vi "Begin.vi"() -> (0 "error out":errorcluster)   [LabVIEW 2013]
doc: "Called before other user functions, this VI is expected to open initial I/O refnums, load in file data, and do all program initialization. Notice that the <B>error out</B> terminal is simply used for data flow. Wiring it to other structures or subVIs ensures that this VI runs first."
uses:
  <vilib>/Rock Robotics/WPI/DriverStation/WPI_DriverStationRobotMode2.ctl
  <vilib>/Rock Robotics/WPI/Joystick/WPI_JoystickDeviceEnum.ctl
  <vilib>/Rock Robotics/WPI/SafetyOutput/WPI_SafetyOutputConfigMenu.ctl
  <vilib>/Rock Robotics/WPI/CAN/Jaguar/SubVIs/WPI_CANJaguar_ControlMode.ctl
  <vilib>/Rock Robotics/WPI/CAN/Jaguar/SubVIs/WPI_CANJaguar_PositionReference.ctl
  Robot Global Data.vi
  <vilib>/Utility/config.llb/Read Key (Double).vi
  <vilib>/Utility/config.llb/Read Key (String).vi
  <vilib>/Rock Robotics/WPI/MotorControl/WPI_MotorControlOpen Jaguar.vi
  <vilib>/Rock Robotics/WPI/RobotDrive/WPI_RobotDriveOpen4MotorWithCANJaguar.vi
  <vilib>/Rock Robotics/WPI/MotorControl/WPI_MotorControlOpenCANJaguar.vi
  <vilib>/Rock Robotics/SystemInterfaces/Typedef/FPGA_TypedefDigitalModule.ctl
  <vilib>/Utility/config.llb/NI_LVConfig.lvlib
  <vilib>/Rock Robotics/WPI/Solenoid/WPI_SolenoidChannel.ctl
  <vilib>/Rock Robotics/SystemInterfaces/DIO/FPGA_DIOChannel.ctl
  <vilib>/Rock Robotics/SystemInterfaces/DIO/FPGA_DIORelayChannel.ctl
  <vilib>/Rock Robotics/WPI/Solenoid/WPI_SolenoidOpenSingle.vi
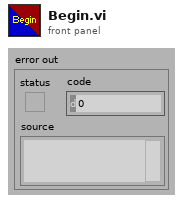
[diagram p1: front panel]
types:
  T1 = typedef "WPI_SafetyOutputConfigMenu.ctl" = enum16{"Enable", "Disable"}
  T2 = typedef "WPI_JoystickDeviceEnum.ctl" = enum16{"USB 1", "USB 2", "USB 3", "USB 4", "Kinect 1", "Kinect 2"}
  T3 = cluster{"Left Motor Positions":cluster{"Low Extreme - 0 Degrees":dbl, "High Extreme - 180 Degrees":dbl}, "Right Motor Positions":cluster{"Low Extreme - 0 Degrees":dbl, "High Extreme - 180 Degrees":dbl}}
  T4 = cluster{"Low Extreme - 0 Degrees":dbl, "High Extreme - 180 Degrees":dbl}
  T5 = typedef "WPI_DriverStationRobotMode2.ctl" = enum16{"Autonomous Disabled", "Autonomous Enabled", "Teleop Disabled", "Teleop Enabled", "Timeout", "Finish", "Test Disabled", "Test Enabled"}
  T6 = typedef "NI_LVConfig.lvlib/Config Data RefNum.ctl" = refnum<k1>
  T7 = typedef "WPI_RobotDriveDevRef.ctl" = cluster{"DevStatus":errorcluster, "Motors[]":T8[], "Square Inputs":bool, "Max Output":dbl, "Isochronous":bool}
  T8 = typedef "WPI_MotorControlDeviceRef.ctl" = cluster{"DeviceStatus":errorcluster, "Type":enum16{"PWM", "CAN"}, "PWM":cluster{"Digital Module":T9, "PWM Channel":T10, "DeadBand":T11}, "CAN":cluster{"Device Number":u8, "Control Mode":T12, "Semaphore":T13, "Max Vout":dbl}, "Invert":bool, "TransformRef":T14, "InvTransformRef":T14}
  T9 = typedef "FPGA_TypedefDigitalModule.ctl" = enum16{"Digital Module 1", "Digital Module 2"}
  T10 = typedef "FPGA_DIOPWMChannel.ctl" = enum8{"PWM 1", "PWM 2", "PWM 3", "PWM 4", "PWM 5", "PWM 6", "PWM 7", "PWM 8", "PWM 9", "PWM 10", "Invalid"}
  T11 = typedef "WPI_PWMDeadband.ctl" = cluster{"Name":string, "maxPositivePwm":i32, "minPositivePwm":i32, "centerPwm":i32, "maxNegativePwm":i32, "minNegativePwm":i32, "angularRange":u16}
  T12 = typedef "WPI_CANJaguar_ControlMode.ctl" = enum8{"Percent VBus", "Current", "Speed", "Position", "Voltage"}
  T13 = typedef "Semaphore RefNum" = refnum<k1>
  T14 = typedef "WPI_PWMTransform_ConPane.ctl" = refnum<vi>
  T15 = typedef "FPGA_DIORelayChannel.ctl" = enum8{"Relay 1", "Relay 2", "Relay 3", "Relay 4", "Relay 5", "Relay 6", "Relay 7", "Relay 8", "Invalid"}
  T16 = typedef "FPGA_DIOChannel.ctl" = enum8{"DIO 1", "DIO 2", "DIO 3", "DIO 4", "DIO 5", "DIO 6", "DIO 7", "DIO 8", "DIO 9", "DIO 10", "DIO 11", "DIO 12", "DIO 13", "DIO 14", "Invalid"}
  T17 = typedef "WPI_SolenoidChannel.ctl" = enum8{"Solenoid 1", "Solenoid 2", "Solenoid 3", "Solenoid 4", "Solenoid 5", "Solenoid 6", "Solenoid 7", "Solenoid 8", "Invalid"}
  T18 = typedef "WPI_SolenoidDevRef.ctl" = cluster{"DevStatus":errorcluster, "Solenoid Module":T19, "Forward Solenoid Channel":T17, "Reverse Solenoid Channel":T17}
  T19 = typedef "FPGA_TypedefSolenoidModule.ctl" = enum16{"Solenoid Module 1", "Solenoid Module 2"}
  T20 = typedef "WPI_CompressorDevRef.ctl" = cluster{"DevStatus":errorcluster, "DigitalInputDevRef":T21, "RelayDevRef":T22}
  T21 = typedef "WPI_DigitalInputDevRef.ctl" = cluster{"DevStatus":errorcluster, "DIO Channel":T16, "Digital Module":T9}
  T22 = typedef "WPI_RelayDevRef.ctl" = cluster{"DevStatus":errorcluster, "Relay Channel":T15, "Digital Module":T9, "Relay Direction":T23}
  T23 = typedef "WPI_RelayDirection.ctl" = enum16{"Both directions", "Forward only", "Reverse only"}
  T24 = typedef "WPI_CANJaguar_PositionReference.ctl" = u8
  T25 = typedef "WPI_JoystickDevRef.ctl" = cluster{"Device":T2}
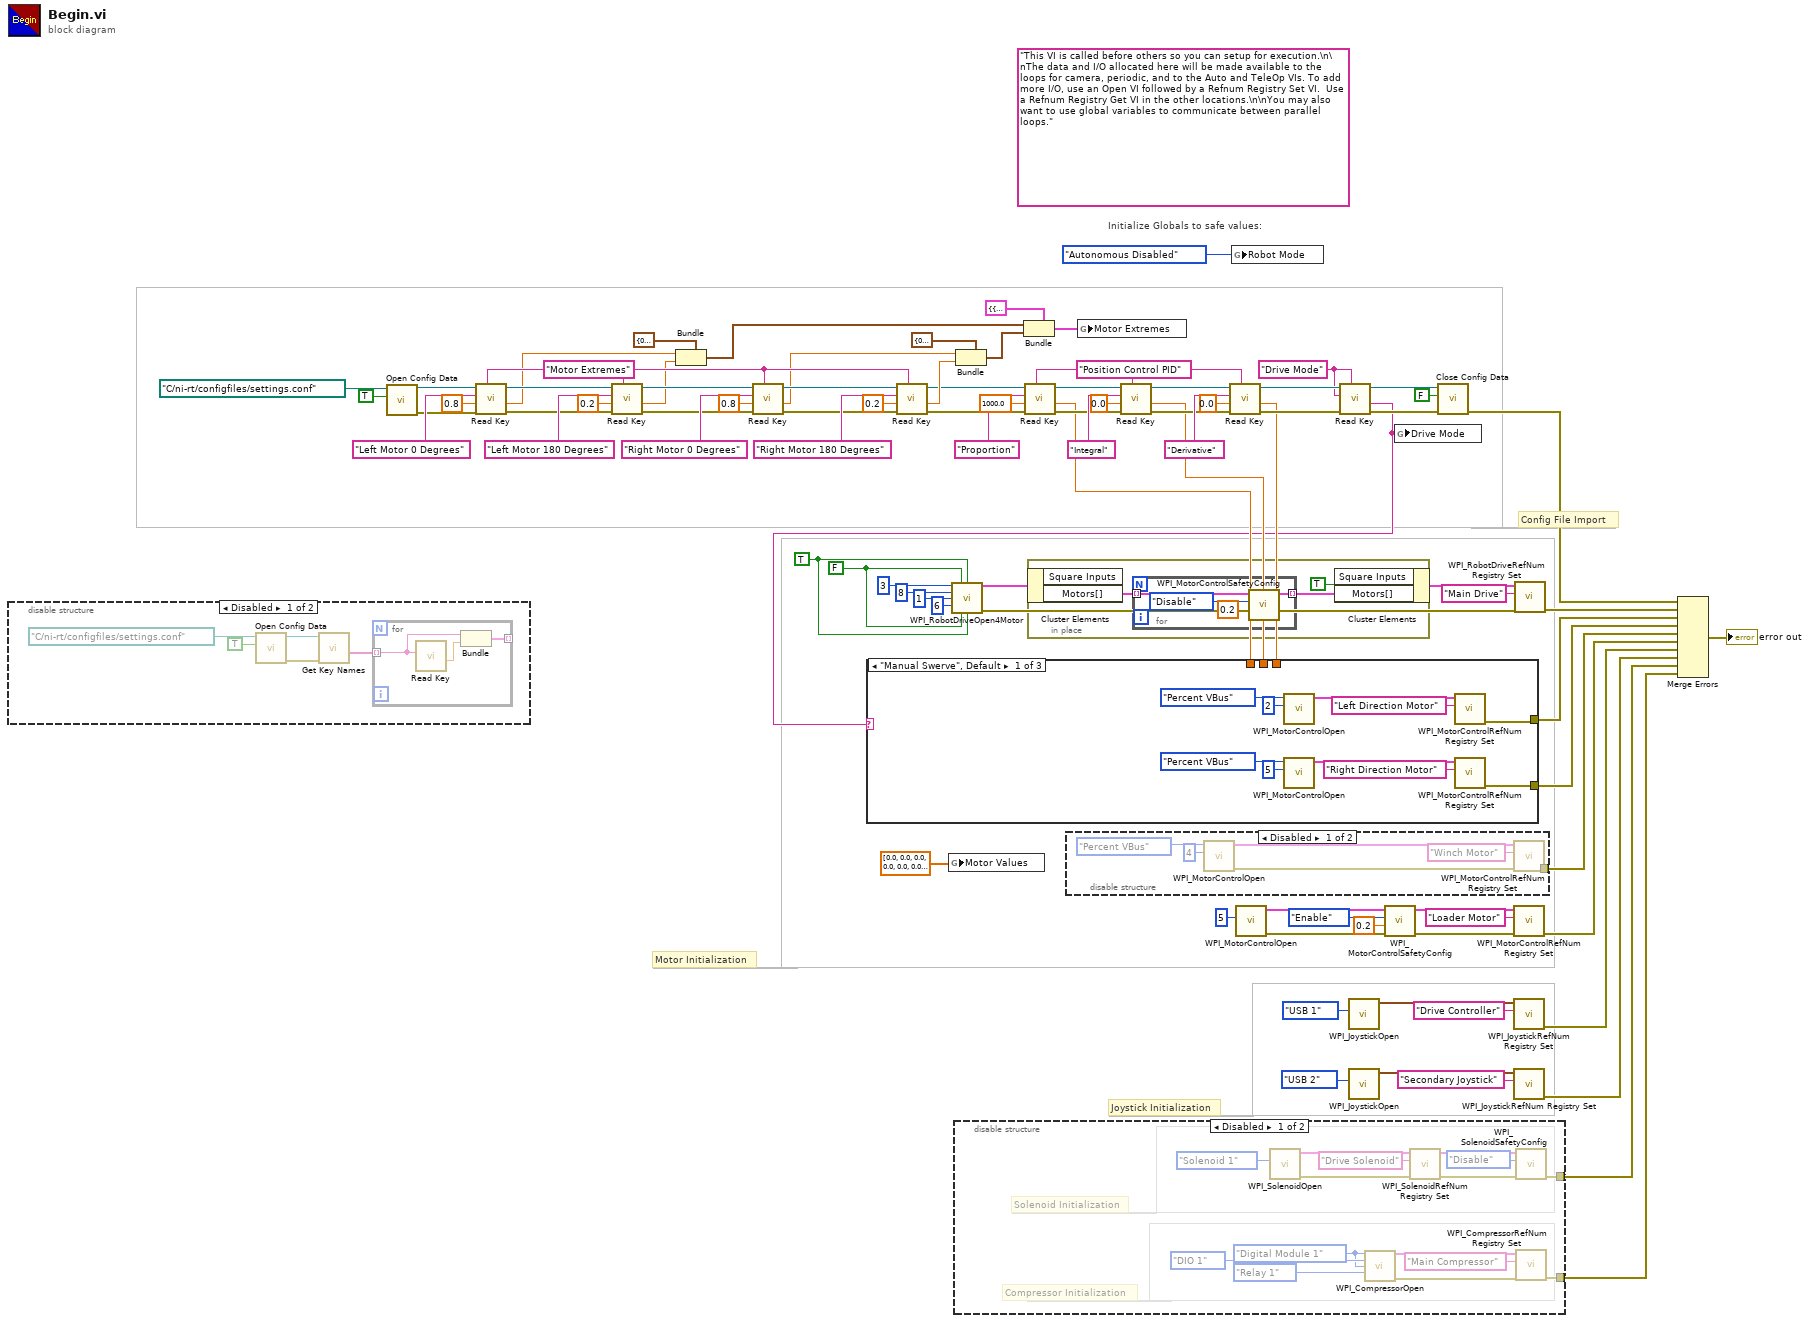
[diagram p0: block diagram]
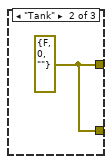
[diagram p5: hidden frame]
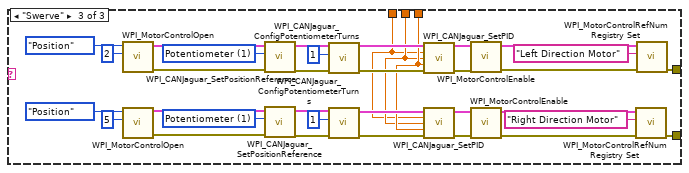
[diagram p6: hidden frame]
diagram:
  w1 = TRUE ("Rear Right Motor Inverted")
  w2 = FALSE
  w27 = "Drive Mode" ("section")
  w56 = "Position Control PID" ("section")
  w70 = "Motor Extremes" ("section")
  (unwired) "This VI is called before others so you can setup for execution.\n\nThe data and I/O allocated here will be made available to the loops for camera, periodic, and to the Auto and TeleOp VIs. To add more I/O, use an Open VI followed by a Refnum Registry Set VI.  Use a Refnum Registry Get VI in the other locations.\n\nYou may also want to use global variables to communicate between parallel loops."
  # "Config File Import"
  # "Joystick Initialization"
  # "Motor Initialization"
  # "Initialize Globals to safe values:"
  n1 = disable-structure shown="Disabled" {
    frame Disabled {
      n2 = call <vilib>:"Open Config Data.vi"("create file if necessary (T)"=TRUE, "configuration file path"=path "C:/ni-rt/configfiles/settings.conf") -> ("error out"=w91:errorcluster, "refnum"=w92:T6)  [unwired: 7 in, 1 out]
      n3 = call <vilib>:"Get Key Names.vi"("error in (no error)"=w91, "refnum"=w92) -> ("key names"=w90:string[])  [unwired: 6 in, 3 out]
      n4 = for {
        tunnel: w90 -> [w97] mode=indexing
        tunnel: [w95] -> _ mode=indexing
        n5 = call-poly <vilib>:"Read Key.vi"("key"=w97) -> ("value"=w96:dbl)  [unwired: 7 in, 3 out]
        n6 = Bundle("String"=w97, "value"=w96) -> (w95:cluster{"String":string, "value":dbl})  [unwired: 1 in]
      }
    }
    frame Enabled {
    }
  }
  n7 = call <vilib>:"Open Config Data.vi"("create file if necessary (T)"=TRUE, "configuration file path"=path "C:/ni-rt/configfiles/settings.conf") -> ("error out"=w34:errorcluster, "refnum"=w83:T6)  [unwired: 7 in, 1 out]
  n8 = call-poly <vilib>:"Read Key.vi"("section"=w70, "error in (no error)"=w34, "default value"=0.8, "key"="Left Motor 0 Degrees", "refnum"=w83) -> ("error out"=w35:errorcluster, "value"=w55:dbl, "refnum out"=w78:T6)  [unwired: 3 in, 1 out]
  n9 = call-poly <vilib>:"Read Key.vi"("section"=w70, "error in (no error)"=w35, "default value"=0.2, "key"="Left Motor 180 Degrees", "refnum"=w78) -> ("error out"=w36:errorcluster, "value"=w54:dbl, "refnum out"=w72:T6)  [unwired: 3 in, 1 out]
  n10 = Bundle(cluster=T4 {"Low Extreme - 0 Degrees"=0.0, "High Extreme - 180 Degrees"=0.0} ("Left Motor Positions"), "Low Extreme - 0 Degrees"=w55, "High Extreme - 180 Degrees"=w54) -> (w65:T4)
  n11 = call-poly <vilib>:"Read Key.vi"("section"=w70, "error in (no error)"=w36, "default value"=0.8, "key"="Right Motor 0 Degrees", "refnum"=w72) -> ("error out"=w37:errorcluster, "value"=w53:dbl, "refnum out"=w73:T6)  [unwired: 3 in, 1 out]
  n12 = call-poly <vilib>:"Read Key.vi"("section"=w70, "error in (no error)"=w37, "default value"=0.2, "key"="Right Motor 180 Degrees", "refnum"=w73) -> ("error out"=w38:errorcluster, "value"=w52:dbl, "refnum out"=w51:T6)  [unwired: 3 in, 1 out]
  n13 = global write "Robot Global Data.vi" "Motor Values"(dbl[] [0.0, 0.0, 0.0, 0.0, 0.0, 0.0, 0.0, 0.0]) -> ()
  n14 = call-poly <vilib>:"WPI_RobotDriveOpen4Motor.vi"("Rear Left Motor"=u8 3, "Rear Left Motor Inverted"=w2, "Rear Right Motor Inverted"=w1, "Rear Right Motor"=u8 8, "Front Left Motor"=u8 1, "Front Right Motor"=u8 6, "Front Left Motor Inverted"=w2, "Front Right Motor Inverted"=w1) -> ("RobotDriveDevRef"=w49:T7, "error out"=w41:errorcluster)  [unwired: 6 in]
  n15 = disable-structure shown="Disabled" {
    disable-tunnel: [w105 _] -> w24
    disable-tunnel: [w104 _] -> w20
    frame Disabled {
      w99 = FPGA_TypedefDigitalModule."Digital Module 1" ("Pressure Switch Digital Module (Module 1)")
      # "Compressor Initialization"
      # "Solenoid Initialization"
      n16 = call-poly <vilib>:"WPI_SolenoidOpen.vi"("Solenoid Channel"=WPI_SolenoidChannel."Solenoid 1") -> ("error out"=w111:errorcluster, "SolenoidDevRef"=w112:T18)  [unwired: 9 in]
      n17 = call <vilib>:"WPI_CompressorOpen.vi"("Pressure Switch Digital Module (Module 1)"=w99, "Pressure Switch DIO Channel"=FPGA_DIOChannel."DIO 1", "Relay Digital Module (Module 1)"=w99, "Relay Channel"=FPGA_DIORelayChannel."Relay 1") -> ("CompressorDevRef"=w103:T20, "error out"=w98:errorcluster)  [unwired: 10 in]
      n18 = call <vilib>:"WPI_SolenoidRefNum Registry Set.vi"("error in (no error)"=w111, "refnum name"="Drive Solenoid", "SolenoidDevRef"=w112) -> ("error out"=w109:errorcluster, "SolenoidDevRef"=w110:T18)  [unwired: 7 in]
      n19 = call <vilib>:"WPI_SolenoidSafetyConfig.vi"("error in (no error)"=w109, "mode"=WPI_SafetyOutputConfigMenu."Disable", "SolenoidDevRef"=w110) -> ("error out"=w105:errorcluster)  [unwired: 7 in, 1 out]
      n20 = call <vilib>:"WPI_CompressorRefNum Registry Set.vi"("error in (no error)"=w98, "refnum name"="Main Compressor", "CompressorDevRef"=w103) -> ("error out"=w104:errorcluster)  [unwired: 7 in, 1 out]
    }
    frame Enabled {
    }
  }
  n21 = Bundle(cluster=T4 {"Low Extreme - 0 Degrees"=0.0, "High Extreme - 180 Degrees"=0.0} ("Right Motor Positions"), "Low Extreme - 0 Degrees"=w53, "High Extreme - 180 Degrees"=w52) -> (w66:T4)
  n22 = Bundle(cluster=T3 {"Left Motor Positions"={"Low Extreme - 0 Degrees"=0.0, "High Extreme - 180 Degrees"=0.0}, "Right Motor Positions"={"Low Extreme - 0 Degrees"=0.0, "High Extreme - 180 Degrees"=0.0}} ("Motor Extremes"), "Left Motor Positions"=w65, "Right Motor Positions"=w66) -> (w50:T3)
  n23 = call-poly <vilib>:"Read Key.vi"("section"=w56, "error in (no error)"=w38, "default value"=1000.0, "key"="Proportion", "refnum"=w51) -> ("error out"=w39:errorcluster, "value"=w17:dbl, "refnum out"=w60:T6)  [unwired: 3 in, 1 out]
  n24 = in-place {
    n25 = in-place-cluster #1(w49) -> ("Motors[]"=w114:T8[])  [unwired: 1 out]
    n26 = for {
      tunnel: w114 -> [w119] mode=indexing
      tunnel: [w118] -> w113 mode=indexing
      n27 = call <vilib>:"WPI_MotorControlSafetyConfig.vi"("timeout (s)"=0.2, "mode"=WPI_SafetyOutputConfigMenu."Disable", "MotorControlDevRef"=w119) -> ("MotorControlDevRef"=w118:T8)  [unwired: 7 in, 1 out]
    }
    n28 = in-place-cluster #1("Square Inputs"=TRUE, "Motors[]"=w113) -> (w48:T7)
  }
  n29 = disable-structure shown="Disabled" {
    disable-tunnel: [w120 _] -> w32
    frame Disabled {
      n30 = call-poly <vilib>:"WPI_MotorControlOpen.vi"("Device Number"=u8 4, "Control Mode"=WPI_CANJaguar_ControlMode."Percent VBus") -> ("error out"=w121:errorcluster, "MotorControlDeviceRef"=w122:T8)  [unwired: 8 in]
      n31 = call <vilib>:"WPI_MotorControlRefNum Registry Set.vi"("error in (no error)"=w121, "refnum name"="Winch Motor", "MotorControlDevRef"=w122) -> ("error out"=w120:errorcluster)  [unwired: 7 in, 1 out]
    }
    frame Enabled {
    }
  }
  n32 = global write "Robot Global Data.vi" "Motor Extremes"(w50) -> ()
  n33 = call-poly <vilib>:"Read Key.vi"("section"=w56, "error in (no error)"=w39, "default value"=0.0, "key"="Integral", "refnum"=w60) -> ("error out"=w40:errorcluster, "value"=w18:dbl, "refnum out"=w57:T6)  [unwired: 3 in, 1 out]
  n34 = call-poly <vilib>:"Read Key.vi"("section"=w56, "error in (no error)"=w40, "default value"=0.0, "key"="Derivative", "refnum"=w57) -> ("error out"=w30:errorcluster, "value"=w19:dbl, "refnum out"=w31:T6)  [unwired: 3 in, 1 out]
  n35 = global write "Robot Global Data.vi" "Robot Mode"(WPI_DriverStationRobotMode2."Autonomous Disabled" ("Robot Mode")) -> ()
  n36 = call-poly <vilib>:"WPI_MotorControlOpen.vi"("PWM Channel"=u8 5 ("Device Number")) -> ("error out"=w7:errorcluster, "MotorControlDeviceRef"=w10:T8)  [unwired: 9 in]
  n37 = call-poly <vilib>:"Read Key.vi"("section"=w27, "error in (no error)"=w30, "key"=w27, "refnum"=w31) -> ("error out"=w29:errorcluster, "value"=w14:string, "refnum out"=w28:T6)  [unwired: 4 in, 1 out]
  n38 = case shown="\"Manual Swerve\", Default" w14 {
    tunnel: [w126 w136 w141] -> w16
    tunnel: [w127 w136 w140] -> w15
    tunnel: w19 -> [_ _ w139]
    tunnel: w18 -> [_ _ w138]
    tunnel: w17 -> [_ _ w137]
    frame "Manual Swerve", Default {
      n39 = call-poly <vilib>:"WPI_MotorControlOpen.vi"("Device Number"=u8 2, "Control Mode"=WPI_CANJaguar_ControlMode."Percent VBus") -> ("MotorControlDeviceRef"=w130:T8)  [unwired: 8 in, 1 out]
      n40 = call-poly <vilib>:"WPI_MotorControlOpen.vi"("Device Number"=u8 5, "Control Mode"=WPI_CANJaguar_ControlMode."Percent VBus") -> ("MotorControlDeviceRef"=w129:T8)  [unwired: 8 in, 1 out]
      n41 = call <vilib>:"WPI_MotorControlRefNum Registry Set.vi"("refnum name"="Left Direction Motor", "MotorControlDevRef"=w130) -> ("error out"=w126:errorcluster)  [unwired: 8 in, 1 out]
      n42 = call <vilib>:"WPI_MotorControlRefNum Registry Set.vi"("refnum name"="Right Direction Motor", "MotorControlDevRef"=w129) -> ("error out"=w127:errorcluster)  [unwired: 8 in, 1 out]
    }
    frame "Tank" {
      w136 = errorcluster {"status"=FALSE, "code"=0, "source"=""} ("error out")
    }
    frame "Swerve" {
      w151 = T24 1 items=["Quad Encoder"=0, "Potentiometer"=1, "None"=255] ("Position Reference")
      w158 = T24 1 items=["Quad Encoder"=0, "Potentiometer"=1, "None"=255] ("Position Reference")
      n43 = call-poly <vilib>:"WPI_MotorControlOpen.vi"("Device Number"=u8 2, "Control Mode"=WPI_CANJaguar_ControlMode."Position") -> ("error out"=w155:errorcluster, "MotorControlDeviceRef"=w161:T8)  [unwired: 8 in]
      n44 = call-poly <vilib>:"WPI_MotorControlOpen.vi"("Device Number"=u8 5, "Control Mode"=WPI_CANJaguar_ControlMode."Position") -> ("error out"=w146:errorcluster, "MotorControlDeviceRef"=w147:T8)  [unwired: 8 in]
      n45 = call <vilib>:"WPI_CANJaguar_SetPositionReference.vi"("error in (no error)"=w155, "Position Reference"=w158, "CAN Jaguar Ref"=w161) -> ("error out"=w156:errorcluster, "CAN Jaguar Ref Out"=w160:T8)  [unwired: 7 in]
      n46 = call <vilib>:"WPI_CANJaguar_SetPositionReference.vi"("error in (no error)"=w146, "Position Reference"=w151, "CAN Jaguar Ref"=w147) -> ("error out"=w150:errorcluster, "CAN Jaguar Ref Out"=w153:T8)  [unwired: 7 in]
      n47 = call <vilib>:"WPI_CANJaguar_ConfigPotentiometerTurns.vi"("error in (no error)"=w156, "Potentiometer Turns"=u16 1, "CAN Jaguar Ref"=w160) -> ("error out"=w144:errorcluster, "CAN Jaguar Ref Out"=w145:T8)  [unwired: 7 in]
      n48 = call <vilib>:"WPI_CANJaguar_ConfigPotentiometerTurns.vi"("error in (no error)"=w150, "Potentiometer Turns"=u16 1, "CAN Jaguar Ref"=w153) -> ("error out"=w142:errorcluster, "CAN Jaguar Ref Out"=w143:T8)  [unwired: 7 in]
      n49 = call <vilib>:"WPI_CANJaguar_SetPID.vi"("CAN Jaguar Ref"=w145, "P"=w137, "I"=w138, "D"=w139, "error in (no error)"=w144) -> ("CAN Jaguar Ref Out"=w157:T8, "error out"=w154:errorcluster)  [unwired: 9 in]
      n50 = call <vilib>:"WPI_CANJaguar_SetPID.vi"("CAN Jaguar Ref"=w143, "P"=w137, "I"=w138, "D"=w139, "error in (no error)"=w142) -> ("CAN Jaguar Ref Out"=w149:T8, "error out"=w148:errorcluster)  [unwired: 9 in]
      n51 = call <vilib>:"WPI_MotorControlEnable.vi"("error in (no error)"=w154, "CAN Jaguar Ref"=w157) -> ("error out"=w167:errorcluster, "CAN Jaguar Ref Out"=w168:T8)  [unwired: 8 in]
      n52 = call <vilib>:"WPI_MotorControlEnable.vi"("error in (no error)"=w148, "CAN Jaguar Ref"=w149) -> ("error out"=w162:errorcluster, "CAN Jaguar Ref Out"=w163:T8)  [unwired: 8 in]
      n53 = call <vilib>:"WPI_MotorControlRefNum Registry Set.vi"("error in (no error)"=w162, "refnum name"="Right Direction Motor", "MotorControlDevRef"=w163) -> ("error out"=w140:errorcluster)  [unwired: 7 in, 1 out]
      n54 = call <vilib>:"WPI_MotorControlRefNum Registry Set.vi"("error in (no error)"=w167, "refnum name"="Left Direction Motor", "MotorControlDevRef"=w168) -> ("error out"=w141:errorcluster)  [unwired: 7 in, 1 out]
    }
  }
  n55 = call <vilib>:"WPI_JoystickOpen.vi"("JoystickDevice"=WPI_JoystickDeviceEnum."USB 1") -> ("JoystickDevRef"=w44:T25)  [unwired: 10 in]
  n56 = call <vilib>:"WPI_JoystickOpen.vi"("JoystickDevice"=WPI_JoystickDeviceEnum."USB 2") -> ("JoystickDevRef"=w47:T25)  [unwired: 10 in]
  n57 = call <vilib>:"WPI_MotorControlSafetyConfig.vi"("error in (no error)"=w7, "timeout (s)"=0.2, "mode"=WPI_SafetyOutputConfigMenu."Enable", "MotorControlDevRef"=w10) -> ("error out"=w8:errorcluster, "MotorControlDevRef"=w9:T8)  [unwired: 6 in]
  n58 = global write "Robot Global Data.vi" "Drive Mode"(w14) -> ()
  n59 = call <vilib>:"Close Config Data.vi"("error in (no error)"=w29, "write file if changed (T)"=FALSE, "refnum"=w28) -> ("error out"=w33:errorcluster)  [unwired: 7 in, 1 out]
  n60 = call <vilib>:"WPI_MotorControlRefNum Registry Set.vi"("error in (no error)"=w8, "refnum name"="Loader Motor", "MotorControlDevRef"=w9) -> ("error out"=w21:errorcluster)  [unwired: 7 in, 1 out]
  n61 = call <vilib>:"WPI_JoystickRefNum Registry Set.vi"("refnum name"="Drive Controller", "JoystickDevRef"=w44) -> ("error out"=w22:errorcluster)  [unwired: 8 in, 1 out]
  n62 = call <vilib>:"WPI_JoystickRefNum Registry Set.vi"("refnum name"="Secondary Joystick", "JoystickDevRef"=w47) -> ("error out"=w23:errorcluster)  [unwired: 8 in, 1 out]
  n63 = call <vilib>:"WPI_RobotDriveRefNum Registry Set.vi"("error in (no error)"=w41, "refnum name"="Main Drive", "RobotDriveDevRef"=w48) -> ("error out"=w87:errorcluster)  [unwired: 7 in, 1 out]
  n64 = Merge Errors(w33, w87, w16, w15, w32, w21, w22, w23, w24, w20) -> (→"error out":errorcluster)
